vi "Autonomous Independent.vi"   [LabVIEW 2015]
doc: "This VI is called when autonomous begins, and will automatically be terminated when autonomous ends. You can carry out timed or sensor driven robot movement independently without needing to return to the caller."
uses:
  <vilib>/Rock Robotics/WPI/SafetyOutput/WPI_SafetyOutputConfigMenu.ctl
  <vilib>/Rock Robotics/Network Tables/NT Read String.vi
  <vilib>/Rock Robotics/WPI/Utilities/WPI_GetSetVariantRefNum.vi
  <vilib>/addons/control/pid/pid.llb/PID (DBL).vi
  <vilib>/Rock Robotics/WPI/Solenoid/Deprecated/WPI_SolenoidSetBool.vi
  Z navX/navX Library v2/navX Library v2.lvlib
  <vilib>/addons/control/pid/NI_PID_pid.lvlib
panel:
  # "Be sure to right-click and choose Data Operations>>Make Current Value default if you want to save the array values with the VI"
types:
  T1 = cluster{"proportional gain (Kc)":dbl, "integral time (Ti, min)":dbl, "derivative time (Td, min)":dbl}
  T2 = typedef "WPI_SafetyOutputConfigMenu.ctl" = enum16{"Enable", "Disable"}
  T3 = typedef "navX Library v2.lvlib/Z900_navX_DeviceTypeDef.ctl" = cluster{"Interface":cluster{"Protocol":T4, "Update Rate (4Hz-60Hz)":u8, "navX Open TypeDef":variant}, "Notify Packet":refnum<notifier>, "Loop VI Refnum":refnum<vi>, "Ready to Close Occurrence Refnum":refnum<k4>}
  T4 = typedef "navX Library v2.lvlib/Z900_navX_ProtocolTypeDef.ctl" = enum16{"SERIAL", "I2C", "SPI"}
  T5 = cluster{"LinearAcceleration X":dbl, "LinearAcceleration Y":dbl, "LinearAcceleration Z":dbl}
  T6 = cluster{"Velocity X":dbl, "Velocity Y":dbl, "Velocity Z":dbl, "Displacement X":dbl, "Displacement Y":dbl, "Displacement Z":dbl}
  T7 = typedef "WPI_RobotDriveDevRef.ctl" = cluster{"DevStatus":errorcluster, "Motors[]":T8[], "Square Inputs":bool, "Max Output":dbl}
  T8 = typedef "WPI_MotorControlDeviceRef.ctl" = cluster{"DeviceStatus":errorcluster, "Type":T9, "PWM":cluster{"PWM Channel":T10, "DeadBand":T11}, "CAN":cluster{"Device Number":u8, "Control Mode":T12, "Semaphore":T13, "Max Vout":dbl, "TalonSRX Control Mode":T14}, "Invert":bool}
  T9 = typedef "WPI_MotorControlType.ctl" = enum16{"PWM", "CAN", "CANTalonSRX"}
  T10 = typedef "FPGA_DIOPWMChannel.ctl" = enum8{"PWM 0", "PWM 1", "PWM 2", "PWM 3", "PWM 4", "PWM 5", "PWM 6", "PWM 7", "PWM 8", "PWM 9", "PWM MXP 0", "PWM MXP 1", "PWM MXP 2", "PWM MXP 3", "PWM MXP 4", "PWM MXP 5", "PWM MXP 6", "PWM MXP 7", "PWM MXP 8", "PWM MXP 9", "Invalid"}
  T11 = typedef "WPI_PWMDeadband.ctl" = cluster{"Name":string, "maxPositivePwm":i32, "minPositivePwm":i32, "centerPwm":i32, "maxNegativePwm":i32, "minNegativePwm":i32, "angularRange":u16}
  T12 = typedef "WPI_CANJaguar_ControlMode.ctl" = enum8{"Percent VBus", "Current", "Speed", "Position", "Voltage"}
  T13 = typedef "Semaphore RefNum" = refnum<k1>
  T14 = typedef "WPI_CANTalonSRX_APIControlMode.ctl" = enum8{"Percent VBus", "Speed", "Position", "Slave", "Unchanged / Invalid", "Voltage Compensation", "Current", "Motion Profile"}
  T15 = cluster{"Yaw":dbl, "Roll":dbl, "Pitch":dbl, "Heading":dbl, "Fused Heading":dbl}
  T16 = typedef "WPI_SolenoidDevRef.ctl" = cluster{"DevStatus":errorcluster, "Pneumatics Control Module":u8, "Forward Solenoid Channel":T17, "Reverse Solenoid Channel":T17}
  T17 = typedef "WPI_SolenoidChannel.ctl" = enum8{"Solenoid 0", "Solenoid 1", "Solenoid 2", "Solenoid 3", "Solenoid 4", "Solenoid 5", "Solenoid 6", "Solenoid 7", "Invalid"}
  T18 = typedef "WPI_CANTalonSRX_GlobalStatus.ctl" = cluster{"Applied Throttle":dbl, "Module Enabled":bool, "CAN Error":errorcluster, "Closed Loop Error":dbl, "Forward Limit Switch Closed":bool, "Reverse Limit Switch Closed":bool, "Sensor Position":dbl, "Sensor Velocity":dbl, "Current":dbl, "Sticky Fault - Over Temp":bool, "Sticky Fault - Under Voltage":bool, "Sticky Fault - Forward Limit":bool, "Sticky Fault - Reverse Limit":bool, "Sticky Fault - Forward Soft Limit":bool, "Sticky Fault - Reverse Soft Limit":bool, "Brake is Enabled":bool, "Encoder Position":dbl, "Encoder Velocity":dbl, "Encoder Index Count":dbl, "Encoder A Pin State":bool, "Encoder B Pin State":bool, "Encoder Index Pin State":bool, "Analog In":dbl, "Analog In Velocity":dbl, "Temperature (C)":dbl, "Battery Voltage":dbl, "Control 5 Is Supported":bool, "Current Profile Slot Select":dbl, "Pos Div 8":bool, "Vel Div 4":bool, "Pulse Width Position":i32, "Pulse Width Velocity":i32, "Pulse Width Rise To Rise (us)":i32, "Pulse Width Rise To Fall (us)":i32, "Mot Prof Active Is Under Run":bool, "Mot Prof Active Has Under Run":bool, "Mot Prof Active Is Last":bool, "Mot Prof Active Velocity Only":bool, "Mot Prof Active Is Valid":bool, "Mot Prof Buffer Is Full":bool, "Mot Prof Active Profile Slot Select":i32, "Mot Prof NextID":i32, "Mot Prof Count":i32, "Mot Prof Active Velocity":dbl, "Mot Prof Active Position":dbl, "Mot Prof Output Enable":i32}
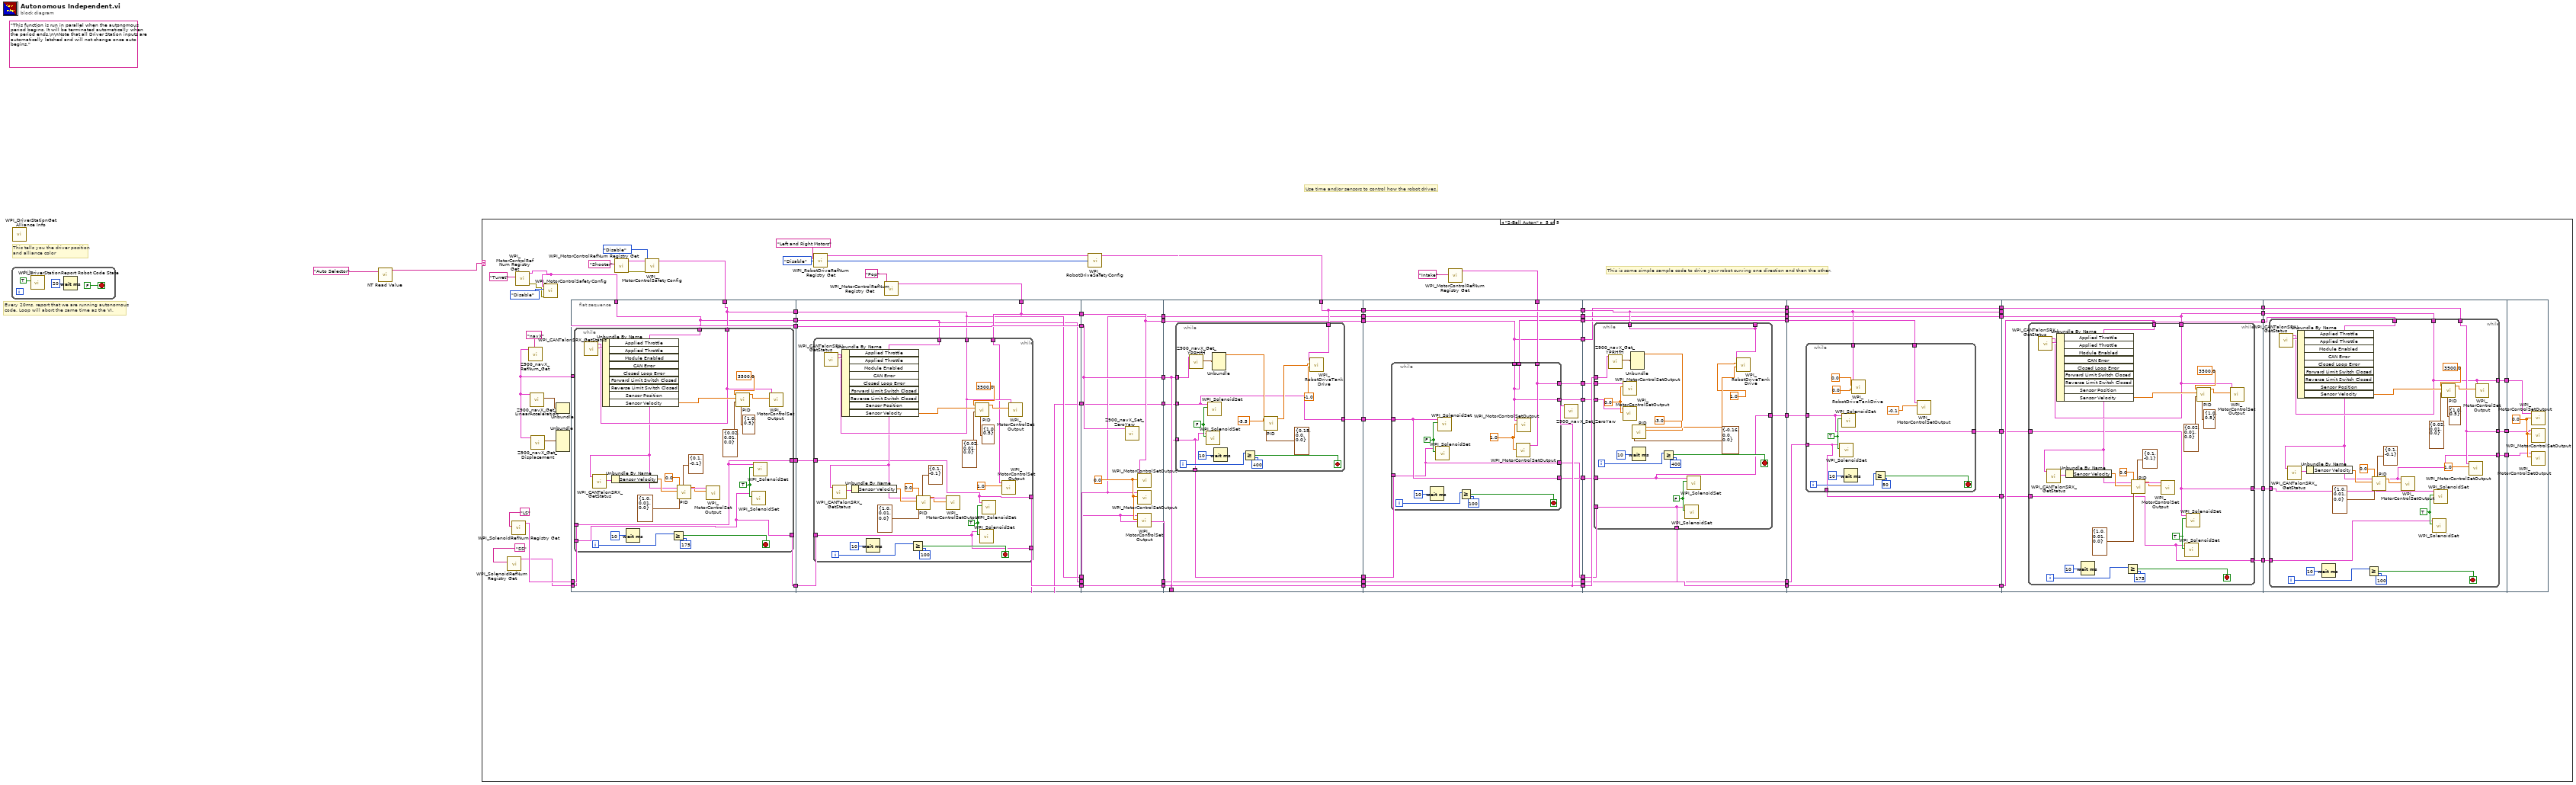
[diagram p0: block diagram]
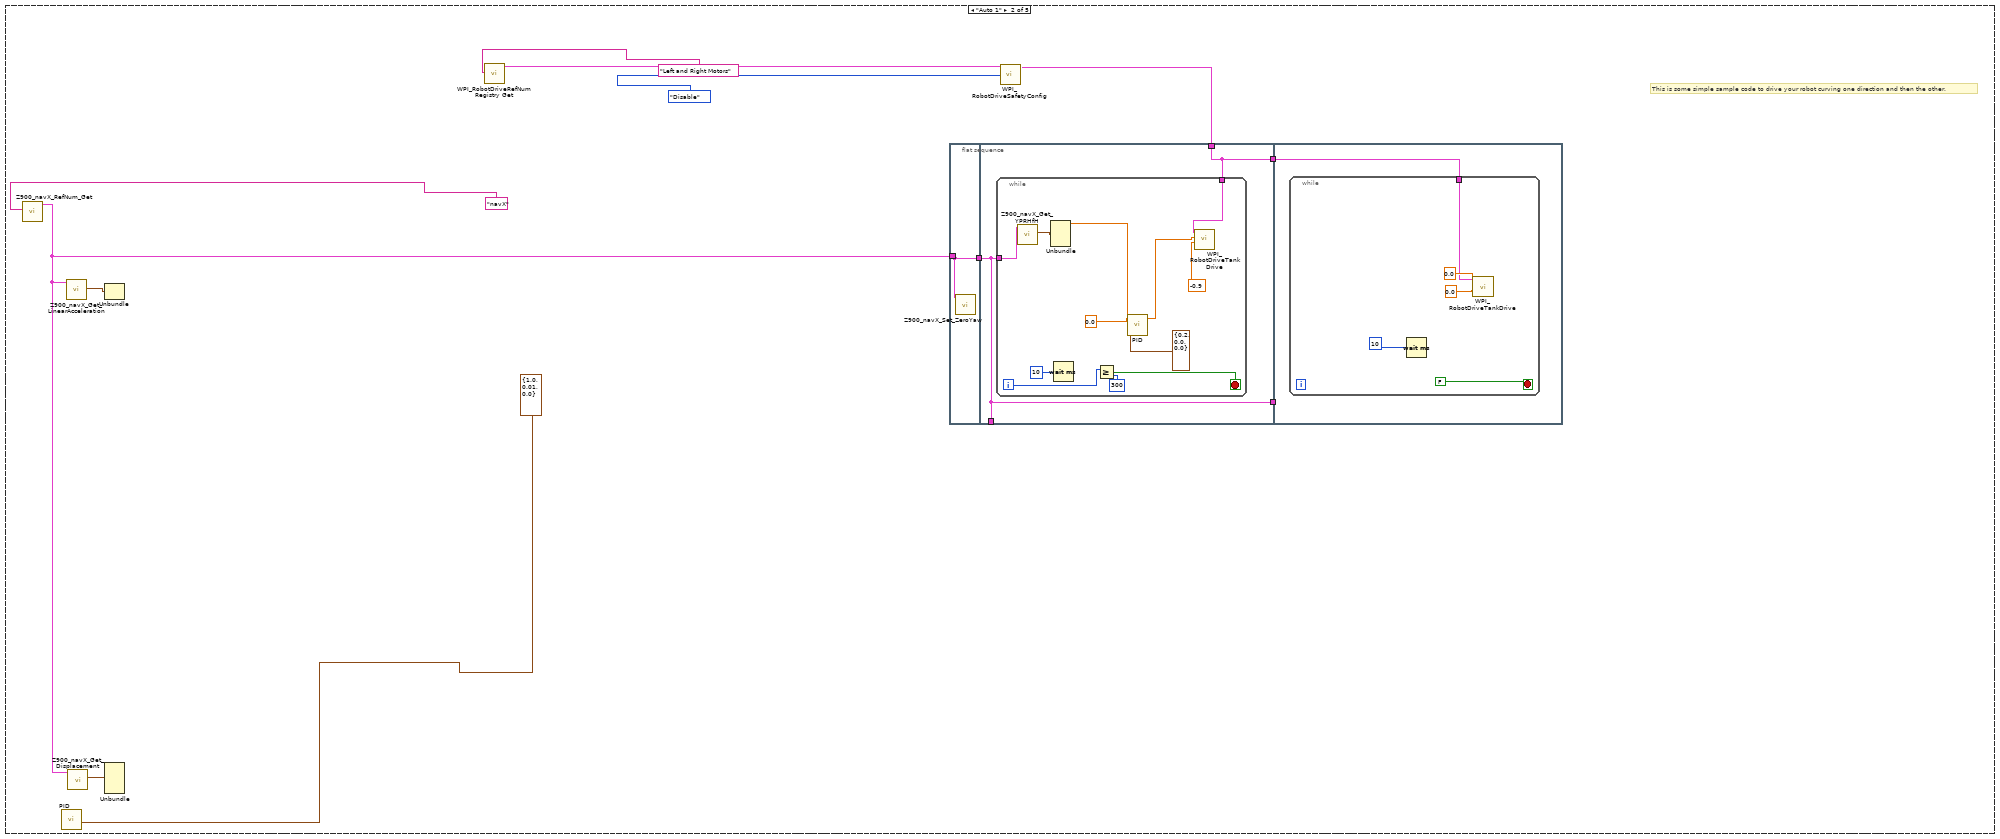
[diagram p3: hidden frame]
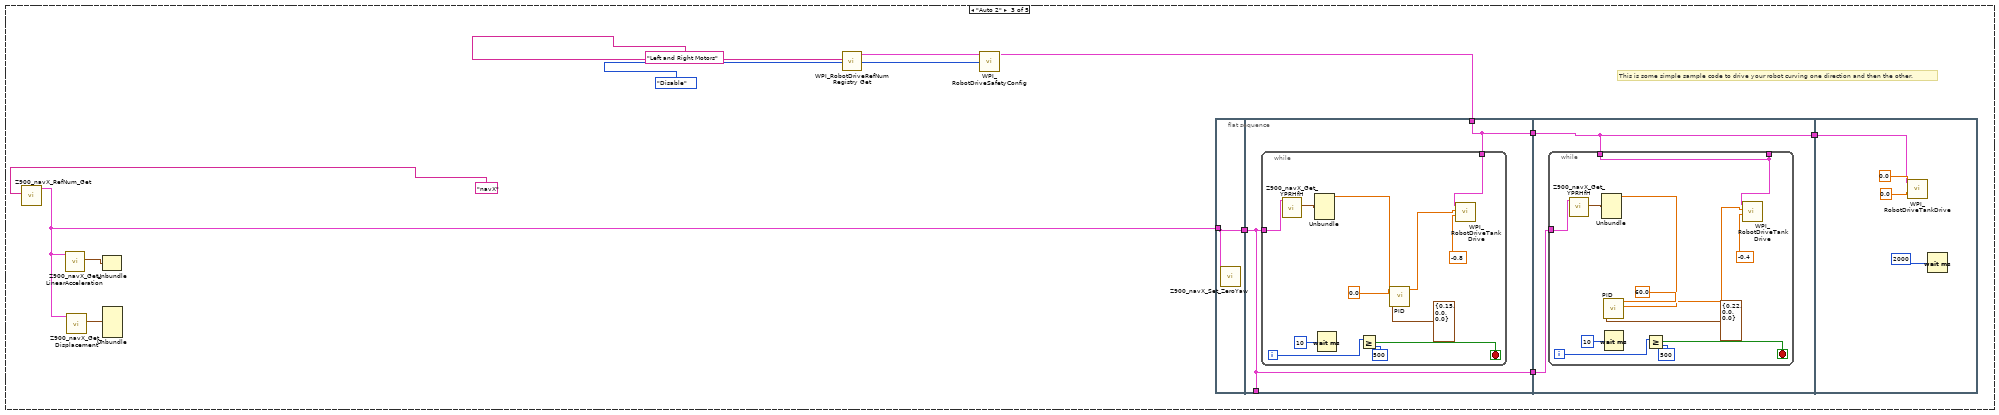
[diagram p4: hidden frame]
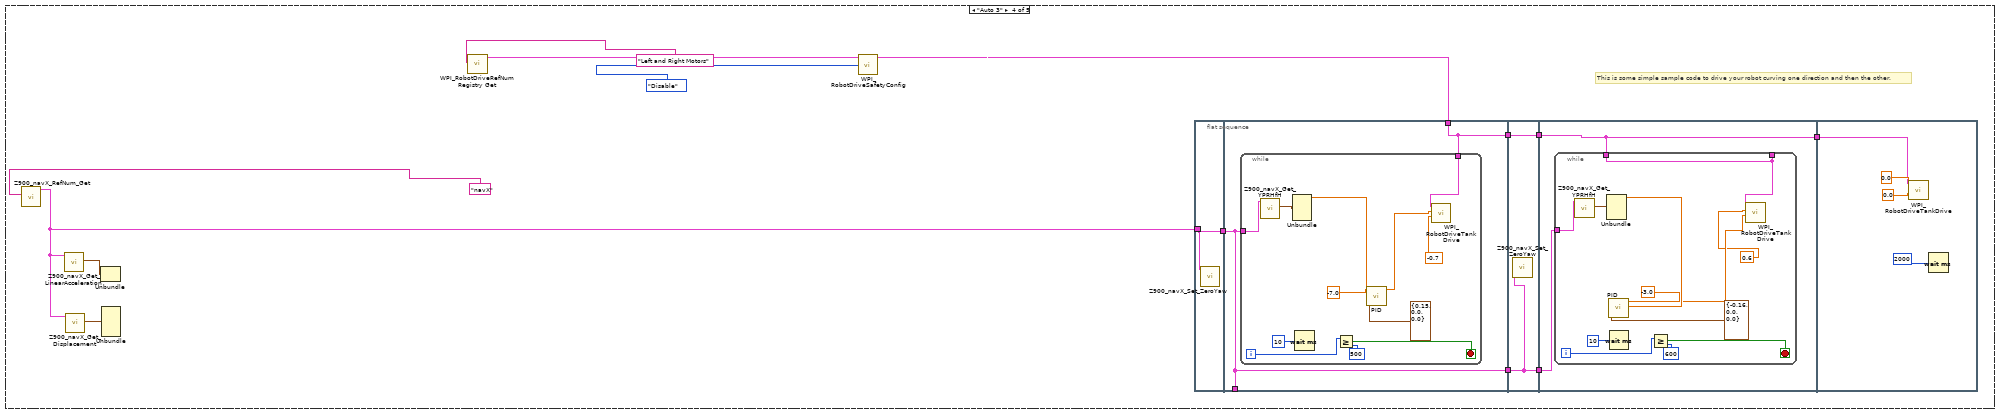
[diagram p5: hidden frame]
diagram:
  (unwired) "This function is run in parallel when the autonomous period begins. It will be terminated automatically when the period ends.\n\nNote that all Driver Station inputs are automatically latched and will not change once auto begins."
  # "Use time and/or sensors to control how the robot drives."
  # "Every 20ms, report that we are running autonomous\ncode. Loop will abort the same time as the VI."
  # "This tells you the driver position\nand alliance color"
  n1 = while {
    stop <- FALSE stop-if-true
    n2 = call <vilib>:"WPI_DriverStationReport Robot Code State.vi"("Autonomous"=TRUE) -> ()  [unwired: 10 in, 1 out]
    n3 = Wait (ms)(milliseconds to wait=u32 20) -> ()  [unwired: 1 out]
  }
  n4 = call <vilib>:"WPI_DriverStationGet Alliance Info.vi"() -> ()  [unwired: 12 out]
  n5 = call-poly <vilib>:"NT Read Value.vi"("Name"="Auto Selector") -> ("String"=w1:string)  [unwired: 9 in, 1 out]
  n6 = case shown="\"2-Ball Auton\"" w1 {
    frame Default {
      # "You can put your main auto here, or you can right-click on the case and make any\nother frame be the default case."
      # "This is the frame that will execute if no selection is made, or if it is not recognized"
    }
    frame "Auto 1" {
      # "This is some simple sample code to drive your robot curving one direction and then the other."
      n7 = call "Z900_navX_RefNum_Get.vi"("refnum name"="navX") -> ("navX Device"=w9:T3)  [unwired: 9 in, 1 out]
      n8 = call-poly <vilib>:"PID.vi"("PID gains"=T1 {"proportional gain (Kc)"=1.0, "integral time (Ti, min)"=0.01, "derivative time (Td, min)"=0.0}) -> ()  [unwired: 9 in, 2 out]
      n9 = call "Z900_navX_Get_LinearAcceleration.vi"("navX Device"=w9) -> ("Linear Acceleration"=w11:T5)  [unwired: 7 in, 3 out]
      n10 = call "Z900_navX_Get_Displacement.vi"("navX Device"=w9) -> ("Displacement"=w10:T6)  [unwired: 7 in, 3 out]
      n11 = Unbundle(w11) -> ()  [unwired: 3 out]
      n12 = Unbundle(w10) -> ()  [unwired: 6 out]
      n13 = call <vilib>:"WPI_RobotDriveRefNum Registry Get.vi"("refnum name"="Left and Right Motors") -> ("RobotDriveDevRef"=w14:T7)  [unwired: 9 in, 1 out]
      n14 = flat-sequence {
        tunnel: w9 -> [w18]
        tunnel: [w18] -> w7
        tunnel: w13 -> [w20]
        tunnel: [w20] -> w17
        tunnel: w7 -> [w19]
        tunnel: [w19] -> _
        tunnel: [w19] -> w6
        tunnel: w17 -> [w33]
        tunnel: w6 -> [_]
        frame #0 {
          n15 = call "Z900_navX_Set_ZeroYaw.vi"("navX Device"=w18) -> ()  [unwired: 9 in, 2 out]
        }
        frame #1 {
          n16 = while {
            tunnel: w20 -> [w29]
            tunnel: w19 -> [w24]
            i -> [w28]
            stop <- w26 stop-if-true
            n17 = call "Z900_navX_Get_YPRHfH.vi"("navX Device"=w24) -> ("YRPHfH"=w25:T15)  [unwired: 7 in, 3 out]
            n18 = Unbundle(w25) -> ("Yaw"=w21:dbl)  [unwired: 4 out]
            n19 = Wait (ms)(milliseconds to wait=10) -> ()  [unwired: 1 out]
            n20 = Greater Or Equal?(x=w28, y=300) -> (x >= y?=w26:bool)
            n21 = call-poly <vilib>:"PID.vi"("PID gains"=T1 {"proportional gain (Kc)"=0.2, "integral time (Ti, min)"=0.0, "derivative time (Td, min)"=0.0}, "process variable"=w21, "setpoint"=0.0) -> ("output"=w22:dbl)  [unwired: 7 in, 1 out]
            n22 = call <vilib>:"WPI_RobotDriveTankDrive.vi"("Right axis value"=-0.9, "Left axis value"=w22, "RobotDriveDevRef"=w29) -> ()  [unwired: 6 in, 3 out]
          }
        }
        frame #2 {
          n23 = while {
            tunnel: w33 -> [w35]
            stop <- FALSE stop-if-true
            n24 = Wait (ms)(milliseconds to wait=10) -> ()  [unwired: 1 out]
            n25 = call <vilib>:"WPI_RobotDriveTankDrive.vi"("Right axis value"=0.0, "Left axis value"=0.0, "RobotDriveDevRef"=w35) -> ()  [unwired: 6 in, 3 out]
          }
        }
      }
      n26 = call <vilib>:"WPI_RobotDriveSafetyConfig.vi"("mode"=WPI_SafetyOutputConfigMenu."Disable", "RobotDriveDevRef"=w14) -> ("RobotDriveDevRef"=w13:T7)  [unwired: 8 in, 1 out]
    }
    frame "Auto 2" {
      # "This is some simple sample code to drive your robot curving one direction and then the other."
      n27 = call "Z900_navX_RefNum_Get.vi"("refnum name"="navX") -> ("navX Device"=w39:T3)  [unwired: 9 in, 1 out]
      n28 = call "Z900_navX_Get_LinearAcceleration.vi"("navX Device"=w39) -> ("Linear Acceleration"=w41:T5)  [unwired: 7 in, 3 out]
      n29 = call "Z900_navX_Get_Displacement.vi"("navX Device"=w39) -> ("Displacement"=w40:T6)  [unwired: 7 in, 3 out]
      n30 = Unbundle(w41) -> ()  [unwired: 3 out]
      n31 = Unbundle(w40) -> ()  [unwired: 6 out]
      n32 = call <vilib>:"WPI_RobotDriveRefNum Registry Get.vi"("refnum name"="Left and Right Motors") -> ("RobotDriveDevRef"=w44:T7)  [unwired: 9 in, 1 out]
      n33 = call <vilib>:"WPI_RobotDriveSafetyConfig.vi"("mode"=WPI_SafetyOutputConfigMenu."Disable", "RobotDriveDevRef"=w44) -> ("RobotDriveDevRef"=w43:T7)  [unwired: 8 in, 1 out]
      n34 = flat-sequence {
        tunnel: w39 -> [w51]
        tunnel: [w51] -> w50
        tunnel: w43 -> [w53]
        tunnel: [w53] -> w49
        tunnel: w50 -> [w52]
        tunnel: [w52] -> _
        tunnel: [w52] -> w48
        tunnel: w49 -> [w67]
        tunnel: [w67] -> w47
        tunnel: w48 -> [w66]
        tunnel: w47 -> [w80]
        frame #0 {
          n35 = call "Z900_navX_Set_ZeroYaw.vi"("navX Device"=w51) -> ()  [unwired: 9 in, 2 out]
        }
        frame #1 {
          n36 = while {
            tunnel: w53 -> [w62]
            tunnel: w52 -> [w57]
            i -> [w61]
            stop <- w59 stop-if-true
            n37 = call "Z900_navX_Get_YPRHfH.vi"("navX Device"=w57) -> ("YRPHfH"=w58:T15)  [unwired: 7 in, 3 out]
            n38 = Unbundle(w58) -> ("Yaw"=w54:dbl)  [unwired: 4 out]
            n39 = Wait (ms)(milliseconds to wait=10) -> ()  [unwired: 1 out]
            n40 = Greater Or Equal?(x=w61, y=500) -> (x >= y?=w59:bool)
            n41 = call-poly <vilib>:"PID.vi"("PID gains"=T1 {"proportional gain (Kc)"=0.15, "integral time (Ti, min)"=0.0, "derivative time (Td, min)"=0.0}, "process variable"=w54, "setpoint"=0.0) -> ("output"=w55:dbl)  [unwired: 7 in, 1 out]
            n42 = call <vilib>:"WPI_RobotDriveTankDrive.vi"("Right axis value"=-0.8, "Left axis value"=w55, "RobotDriveDevRef"=w62) -> ()  [unwired: 6 in, 3 out]
          }
        }
        frame #2 {
          n43 = while {
            tunnel: [w68] -> _
            tunnel: w66 -> [w71]
            tunnel: w67 -> [w68]
            i -> [w76]
            stop <- w74 stop-if-true
            n44 = call "Z900_navX_Get_YPRHfH.vi"("navX Device"=w71) -> ("YRPHfH"=w73:T15)  [unwired: 7 in, 3 out]
            n45 = Unbundle(w73) -> ("Yaw"=w72:dbl)  [unwired: 4 out]
            n46 = call-poly <vilib>:"PID.vi"("PID gains"=T1 {"proportional gain (Kc)"=0.22, "integral time (Ti, min)"=0.0, "derivative time (Td, min)"=0.0}, "process variable"=w72, "setpoint"=60.0) -> ("output"=w69:dbl)  [unwired: 7 in, 1 out]
            n47 = Wait (ms)(milliseconds to wait=10) -> ()  [unwired: 1 out]
            n48 = Greater Or Equal?(x=w76, y=500) -> (x >= y?=w74:bool)
            n49 = call <vilib>:"WPI_RobotDriveTankDrive.vi"("Right axis value"=-0.4, "Left axis value"=w69, "RobotDriveDevRef"=w68) -> ()  [unwired: 6 in, 3 out]
          }
        }
        frame #3 {
          n50 = call <vilib>:"WPI_RobotDriveTankDrive.vi"("Right axis value"=0.0, "Left axis value"=0.0, "RobotDriveDevRef"=w80) -> ()  [unwired: 6 in, 3 out]
          n51 = Wait (ms)(milliseconds to wait=2000) -> ()  [unwired: 1 out]
        }
      }
    }
    frame "Auto 3" {
      # "This is some simple sample code to drive your robot curving one direction and then the other."
      n52 = call "Z900_navX_RefNum_Get.vi"("refnum name"="navX") -> ("navX Device"=w88:T3)  [unwired: 9 in, 1 out]
      n53 = call "Z900_navX_Get_LinearAcceleration.vi"("navX Device"=w88) -> ("Linear Acceleration"=w90:T5)  [unwired: 7 in, 3 out]
      n54 = call "Z900_navX_Get_Displacement.vi"("navX Device"=w88) -> ("Displacement"=w89:T6)  [unwired: 7 in, 3 out]
      n55 = Unbundle(w90) -> ()  [unwired: 3 out]
      n56 = Unbundle(w89) -> ()  [unwired: 6 out]
      n57 = call <vilib>:"WPI_RobotDriveRefNum Registry Get.vi"("refnum name"="Left and Right Motors") -> ("RobotDriveDevRef"=w93:T7)  [unwired: 9 in, 1 out]
      n58 = call <vilib>:"WPI_RobotDriveSafetyConfig.vi"("mode"=WPI_SafetyOutputConfigMenu."Disable", "RobotDriveDevRef"=w93) -> ("RobotDriveDevRef"=w92:T7)  [unwired: 8 in, 1 out]
      n59 = flat-sequence {
        tunnel: w88 -> [w98]
        tunnel: [w98] -> w97
        tunnel: w92 -> [w100]
        tunnel: [w100] -> w87
        tunnel: w97 -> [w99]
        tunnel: [w99] -> _
        tunnel: [w99] -> w85
        tunnel: w87 -> [w114]
        tunnel: [w114] -> w86
        tunnel: w85 -> [w113]
        tunnel: [w113] -> w84
        tunnel: w86 -> [w116]
        tunnel: [w116] -> w96
        tunnel: w84 -> [w115]
        tunnel: w96 -> [w129]
        frame #0 {
          n60 = call "Z900_navX_Set_ZeroYaw.vi"("navX Device"=w98) -> ()  [unwired: 9 in, 2 out]
        }
        frame #1 {
          n61 = while {
            tunnel: w100 -> [w109]
            tunnel: w99 -> [w104]
            i -> [w108]
            stop <- w106 stop-if-true
            n62 = call "Z900_navX_Get_YPRHfH.vi"("navX Device"=w104) -> ("YRPHfH"=w105:T15)  [unwired: 7 in, 3 out]
            n63 = Unbundle(w105) -> ("Yaw"=w101:dbl)  [unwired: 4 out]
            n64 = Wait (ms)(milliseconds to wait=10) -> ()  [unwired: 1 out]
            n65 = Greater Or Equal?(x=w108, y=500) -> (x >= y?=w106:bool)
            n66 = call-poly <vilib>:"PID.vi"("PID gains"=T1 {"proportional gain (Kc)"=0.15, "integral time (Ti, min)"=0.0, "derivative time (Td, min)"=0.0}, "process variable"=w101, "setpoint"=-7.0) -> ("output"=w102:dbl)  [unwired: 7 in, 1 out]
            n67 = call <vilib>:"WPI_RobotDriveTankDrive.vi"("Right axis value"=-0.7, "Left axis value"=w102, "RobotDriveDevRef"=w109) -> ()  [unwired: 6 in, 3 out]
          }
        }
        frame #2 {
          n68 = call "Z900_navX_Set_ZeroYaw.vi"("navX Device"=w113) -> ()  [unwired: 9 in, 2 out]
        }
        frame #3 {
          n69 = while {
            tunnel: [w119] -> _
            tunnel: w115 -> [w120]
            tunnel: w116 -> [w119]
            i -> [w125]
            stop <- w123 stop-if-true
            n70 = call "Z900_navX_Get_YPRHfH.vi"("navX Device"=w120) -> ("YRPHfH"=w122:T15)  [unwired: 7 in, 3 out]
            n71 = Unbundle(w122) -> ("Yaw"=w121:dbl)  [unwired: 4 out]
            n72 = call-poly <vilib>:"PID.vi"("PID gains"=T1 {"proportional gain (Kc)"=-0.16, "integral time (Ti, min)"=0.0, "derivative time (Td, min)"=0.0}, "process variable"=w121, "setpoint"=-3.0) -> ("output"=w118:dbl)  [unwired: 7 in, 1 out]
            n73 = Wait (ms)(milliseconds to wait=10) -> ()  [unwired: 1 out]
            n74 = Greater Or Equal?(x=w125, y=600) -> (x >= y?=w123:bool)
            n75 = call <vilib>:"WPI_RobotDriveTankDrive.vi"("Right axis value"=w118, "Left axis value"=0.6, "RobotDriveDevRef"=w119) -> ()  [unwired: 6 in, 3 out]
          }
        }
        frame #4 {
          n76 = call <vilib>:"WPI_RobotDriveTankDrive.vi"("Right axis value"=0.0, "Left axis value"=0.0, "RobotDriveDevRef"=w129) -> ()  [unwired: 6 in, 3 out]
          n77 = Wait (ms)(milliseconds to wait=2000) -> ()  [unwired: 1 out]
        }
      }
    }
    frame "2-Ball Auton" {
      # "This is some simple sample code to drive your robot curving one direction and then the other."
      n78 = call <vilib>:"WPI_SolenoidRefNum Registry Get.vi"("refnum name"="SS") -> ("SolenoidDevRef"=w149:T16)  [unwired: 9 in, 1 out]
      n79 = call <vilib>:"WPI_SolenoidRefNum Registry Get.vi"("refnum name"="LS") -> ("SolenoidDevRef"=w150:T16)  [unwired: 9 in, 1 out]
      n80 = call <vilib>:"WPI_MotorControlRefNum Registry Get.vi"("refnum name"="Turret") -> ("error out"=w187:errorcluster, "MotorControlDevRef"=w189:T8)  [unwired: 9 in]
      n81 = call "Z900_navX_RefNum_Get.vi"("refnum name"="navX") -> ("navX Device"=w204:T3)  [unwired: 9 in, 1 out]
      n82 = call "Z900_navX_Get_LinearAcceleration.vi"("navX Device"=w204) -> ("Linear Acceleration"=w206:T5)  [unwired: 7 in, 3 out]
      n83 = call "Z900_navX_Get_Displacement.vi"("navX Device"=w204) -> ("Displacement"=w205:T6)  [unwired: 7 in, 3 out]
      n84 = call <vilib>:"WPI_MotorControlSafetyConfig.vi"("error in (no error)"=w187, "mode"=WPI_SafetyOutputConfigMenu."Disable", "MotorControlDevRef"=w189) -> ()  [unwired: 7 in, 2 out]
      n85 = Unbundle(w206) -> ()  [unwired: 3 out]
      n86 = Unbundle(w205) -> ()  [unwired: 6 out]
      n87 = flat-sequence {
        tunnel: w204 -> [w219]
        tunnel: [w219] -> w198
        tunnel: w193 -> [w218]
        tunnel: w189 -> [w217]
        tunnel: [w218] -> w191
        tunnel: [w217] -> w190
        tunnel: w150 -> [w216]
        tunnel: w149 -> [w215]
        tunnel: [w214] -> w148
        tunnel: [w213] -> w147
        tunnel: [w248] -> w199
        tunnel: w198 -> [w248]
        tunnel: w191 -> [w246]
        tunnel: w190 -> [w245]
        tunnel: w185 -> [w247]
        tunnel: [w247] -> w184
        tunnel: [w246] -> w183
        tunnel: [w245] -> w182
        tunnel: w148 -> [w244]
        tunnel: w147 -> [w243]
        tunnel: [w242] -> w145
        tunnel: [w241] -> w143
        tunnel: [w278] -> w212
        tunnel: w199 -> [w278]
        tunnel: w184 -> [w276]
        tunnel: w183 -> [w275]
        tunnel: w182 -> [w274]
        tunnel: [w276] -> w179
        tunnel: [w275] -> w167
        tunnel: [w274] -> w162
        tunnel: [w273] -> w146
        tunnel: w145 -> [w273]
        tunnel: [w272] -> w144
        tunnel: w143 -> [w272]
        tunnel: w208 -> [w287]
        tunnel: [w287] -> w203
        tunnel: w212 -> [w286]
        tunnel: [w286] -> _
        tunnel: [w286] -> w201
        tunnel: [w285] -> w180
        tunnel: w179 -> [w285]
        tunnel: [w284] -> w168
        tunnel: w167 -> [w284]
        tunnel: [w283] -> w163
        tunnel: w162 -> [w283]
        tunnel: w146 -> [w282]
        tunnel: w144 -> [w281]
        tunnel: [w280] -> w142
        tunnel: [w279] -> w141
        tunnel: w203 -> [w315]
        tunnel: [w315] -> w202
        tunnel: w201 -> [w314]
        tunnel: [w314] -> w200
        tunnel: w180 -> [w307]
        tunnel: w178 -> [w313]
        tunnel: [w312] -> w174
        tunnel: [w311] -> w173
        tunnel: [w310] -> w172
        tunnel: [w309] -> w169
        tunnel: w168 -> [w309]
        tunnel: [w308] -> w164
        tunnel: w163 -> [w308]
        tunnel: [w307] -> w156
        tunnel: w142 -> [w306]
        tunnel: w141 -> [w305]
        tunnel: [w304] -> w140
        tunnel: [w303] -> w139
        tunnel: w202 -> [w337]
        tunnel: [w337] -> w177
        tunnel: w200 -> [w336]
        tunnel: [w335] -> w175
        tunnel: w174 -> [w335]
        tunnel: w173 -> [w334]
        tunnel: w172 -> [w333]
        tunnel: [w332] -> w170
        tunnel: w169 -> [w332]
        tunnel: [w331] -> w165
        tunnel: w164 -> [w331]
        tunnel: [w330] -> w157
        tunnel: w156 -> [w330]
        tunnel: w140 -> [w329]
        tunnel: w139 -> [w328]
        tunnel: [w327] -> w138
        tunnel: [w326] -> w137
        tunnel: w177 -> [w363]
        tunnel: [w363] -> w176
        tunnel: w175 -> [w364]
        tunnel: [w362] -> w171
        tunnel: w170 -> [w362]
        tunnel: [w361] -> w166
        tunnel: w165 -> [w361]
        tunnel: [w360] -> w158
        tunnel: w157 -> [w360]
        tunnel: w138 -> [w359]
        tunnel: w137 -> [w358]
        tunnel: [w357] -> w136
        tunnel: [w356] -> w135
        tunnel: w176 -> [_]
        tunnel: w171 -> [w382]
        tunnel: w166 -> [w383]
        tunnel: [w383] -> w161
        tunnel: [w382] -> w160
        tunnel: [w381] -> w159
        tunnel: w158 -> [w381]
        tunnel: w136 -> [w380]
        tunnel: w135 -> [w379]
        tunnel: [w378] -> w134
        tunnel: [w377] -> w133
        tunnel: w161 -> [w412]
        tunnel: w160 -> [w411]
        tunnel: w159 -> [w410]
        tunnel: [w409] -> w155
        tunnel: [w408] -> w154
        tunnel: [w407] -> w153
        tunnel: w134 -> [w406]
        tunnel: w133 -> [w405]
        tunnel: w155 -> [w438]
        tunnel: w154 -> [w437]
        tunnel: w153 -> [w436]
        frame #0 {
          n88 = while {
            tunnel: w218 -> [w231]
            tunnel: w217 -> [w224]
            tunnel: w216 -> [w220]
            tunnel: w215 -> [w221]
            tunnel: [w221] -> w214
            tunnel: [w220] -> w213
            i -> [w239]
            stop <- w237 stop-if-true
            w222 = TRUE
            n89 = call <vilib>:"WPI_CANTalonSRX_GetStatus.vi"("CAN Talon SRX Ref"=w231) -> ("Talon SRX Status"=w233:T18)  [unwired: 8 in, 2 out]
            n90 = call <vilib>:"WPI_CANTalonSRX_GetStatus.vi"("CAN Talon SRX Ref"=w224) -> ("Talon SRX Status"=w229:T18)  [unwired: 8 in, 2 out]
            n91 = Unbundle By Name(w233) -> ("Sensor Velocity"=w235:dbl)  [unwired: 8 out]
            n92 = Unbundle By Name(w229) -> ("Sensor Velocity"=w228:dbl)
            n93 = Wait (ms)(milliseconds to wait=10) -> ()  [unwired: 1 out]
            n94 = Greater Or Equal?(x=w239, y=175) -> (x >= y?=w237:bool)
            n95 = call-poly <vilib>:"PID.vi"("output range"=cluster{"output high":dbl, "output low":dbl} {"output high"=0.1, "output low"=-0.1}, "PID gains"=T1 {"proportional gain (Kc)"=1.0, "integral time (Ti, min)"=0.01, "derivative time (Td, min)"=0.0}, "process variable"=w228, "setpoint"=0.0) -> ("output"=w223:dbl)  [unwired: 6 in, 1 out]
            n96 = call <vilib>:"WPI_MotorControlSetOutput.vi"("Output"=w223, "MotorControlDevRef"=w224) -> ()  [unwired: 7 in, 3 out]
            n97 = call-poly <vilib>:"PID.vi"("output range"=cluster{"output high":dbl, "output low":dbl} {"output high"=1.0, "output low"=0.5}, "PID gains"=T1 {"proportional gain (Kc)"=0.02, "integral time (Ti, min)"=0.01, "derivative time (Td, min)"=0.0}, "process variable"=w235, "setpoint"=3500.0) -> ("output"=w234:dbl)  [unwired: 6 in, 1 out]
            n98 = call-poly <vilib>:"WPI_SolenoidSet.vi"("Value"=w222, "SolenoidDevRef"=w221) -> ()  [unwired: 1 in, 9 out]
            n99 = call-poly <vilib>:"WPI_SolenoidSet.vi"("Value"=w222, "SolenoidDevRef"=w220) -> ()  [unwired: 1 in, 9 out]
            n100 = call <vilib>:"WPI_MotorControlSetOutput.vi"("Output"=w234, "MotorControlDevRef"=w231) -> ()  [unwired: 7 in, 3 out]
          }
        }
        frame #1 {
          n101 = while {
            tunnel: w246 -> [w262]
            tunnel: w245 -> [w255]
            tunnel: w247 -> [w253]
            tunnel: w244 -> [w250]
            tunnel: w243 -> [w249]
            tunnel: [w250] -> w242
            tunnel: [w249] -> w241
            i -> [w270]
            stop <- w268 stop-if-true
            w251 = TRUE
            n102 = call <vilib>:"WPI_CANTalonSRX_GetStatus.vi"("CAN Talon SRX Ref"=w262) -> ("Talon SRX Status"=w264:T18)  [unwired: 8 in, 2 out]
            n103 = call <vilib>:"WPI_CANTalonSRX_GetStatus.vi"("CAN Talon SRX Ref"=w255) -> ("Talon SRX Status"=w260:T18)  [unwired: 8 in, 2 out]
            n104 = Unbundle By Name(w264) -> ("Sensor Velocity"=w266:dbl)  [unwired: 8 out]
            n105 = Unbundle By Name(w260) -> ("Sensor Velocity"=w259:dbl)
            n106 = Wait (ms)(milliseconds to wait=10) -> ()  [unwired: 1 out]
            n107 = Greater Or Equal?(x=w270, y=100) -> (x >= y?=w268:bool)
            n108 = call-poly <vilib>:"PID.vi"("output range"=cluster{"output high":dbl, "output low":dbl} {"output high"=0.1, "output low"=-0.1}, "PID gains"=T1 {"proportional gain (Kc)"=1.0, "integral time (Ti, min)"=0.01, "derivative time (Td, min)"=0.0}, "process variable"=w259, "setpoint"=0.0) -> ("output"=w254:dbl)  [unwired: 6 in, 1 out]
            n109 = call <vilib>:"WPI_MotorControlSetOutput.vi"("Output"=w254, "MotorControlDevRef"=w255) -> ()  [unwired: 7 in, 3 out]
            n110 = call-poly <vilib>:"PID.vi"("output range"=cluster{"output high":dbl, "output low":dbl} {"output high"=1.0, "output low"=0.5}, "PID gains"=T1 {"proportional gain (Kc)"=0.02, "integral time (Ti, min)"=0.01, "derivative time (Td, min)"=0.0}, "process variable"=w266, "setpoint"=3500.0) -> ("output"=w265:dbl)  [unwired: 6 in, 1 out]
            n111 = call-poly <vilib>:"WPI_SolenoidSet.vi"("Value"=w251, "SolenoidDevRef"=w250) -> ()  [unwired: 1 in, 9 out]
            n112 = call-poly <vilib>:"WPI_SolenoidSet.vi"("Value"=w251, "SolenoidDevRef"=w249) -> ()  [unwired: 1 in, 9 out]
            n113 = call <vilib>:"WPI_MotorControlSetOutput.vi"("Output"=1.0, "MotorControlDevRef"=w253) -> ()  [unwired: 7 in, 3 out]
            n114 = call <vilib>:"WPI_MotorControlSetOutput.vi"("Output"=w265, "MotorControlDevRef"=w262) -> ()  [unwired: 7 in, 3 out]
          }
        }
        frame #2 {
          w277 = 0.0
          n115 = call "Z900_navX_Set_ZeroYaw.vi"("navX Device"=w278) -> ()  [unwired: 9 in, 2 out]
          n116 = call <vilib>:"WPI_MotorControlSetOutput.vi"("Output"=w277, "MotorControlDevRef"=w274) -> ()  [unwired: 7 in, 3 out]
          n117 = call <vilib>:"WPI_MotorControlSetOutput.vi"("Output"=w277, "MotorControlDevRef"=w276) -> ()  [unwired: 7 in, 3 out]
          n118 = call <vilib>:"WPI_MotorControlSetOutput.vi"("Output"=w277, "MotorControlDevRef"=w275) -> ()  [unwired: 7 in, 3 out]
        }
        frame #3 {
          n119 = while {
            tunnel: w287 -> [w299]
            tunnel: w286 -> [w294]
            tunnel: w282 -> [w288]
            tunnel: w281 -> [w289]
            tunnel: [w289] -> w280
            tunnel: [w288] -> w279
            i -> [w298]
            stop <- w296 stop-if-true
            w290 = FALSE
            n120 = call "Z900_navX_Get_YPRHfH.vi"("navX Device"=w294) -> ("YRPHfH"=w295:T15)  [unwired: 7 in, 3 out]
            n121 = call-poly <vilib>:"WPI_SolenoidSet.vi"("Value"=w290, "SolenoidDevRef"=w288) -> ()  [unwired: 1 in, 9 out]
            n122 = call-poly <vilib>:"WPI_SolenoidSet.vi"("Value"=w290, "SolenoidDevRef"=w289) -> ()  [unwired: 1 in, 9 out]
            n123 = Unbundle(w295) -> ("Yaw"=w291:dbl)  [unwired: 4 out]
            n124 = Wait (ms)(milliseconds to wait=10) -> ()  [unwired: 1 out]
            n125 = Greater Or Equal?(x=w298, y=400) -> (x >= y?=w296:bool)
            n126 = call-poly <vilib>:"PID.vi"("PID gains"=T1 {"proportional gain (Kc)"=0.15, "integral time (Ti, min)"=0.0, "derivative time (Td, min)"=0.0}, "process variable"=w291, "setpoint"=-5.5) -> ("output"=w292:dbl)  [unwired: 7 in, 1 out]
            n127 = call <vilib>:"WPI_RobotDriveTankDrive.vi"("Right axis value"=-1.0, "Left axis value"=w292, "RobotDriveDevRef"=w299) -> ()  [unwired: 6 in, 3 out]
          }
        }
        frame #4 {
          n128 = while {
            tunnel: w307 -> [w319]
            tunnel: w313 -> [w320]
            tunnel: [w319] -> w312
            tunnel: [w320] -> w311
            tunnel: [w319] -> w310
            tunnel: w306 -> [w317]
            tunnel: w305 -> [w316]
            tunnel: [w317] -> w304
            tunnel: [w316] -> w303
            i -> [w324]
            stop <- w322 stop-if-true
            w318 = FALSE
            w321 = 1.0
            n129 = Wait (ms)(milliseconds to wait=10) -> ()  [unwired: 1 out]
            n130 = call-poly <vilib>:"WPI_SolenoidSet.vi"("Value"=w318, "SolenoidDevRef"=w316) -> ()  [unwired: 1 in, 9 out]
            n131 = call-poly <vilib>:"WPI_SolenoidSet.vi"("Value"=w318, "SolenoidDevRef"=w317) -> ()  [unwired: 1 in, 9 out]
            n132 = Greater Or Equal?(x=w324, y=100) -> (x >= y?=w322:bool)
            n133 = call <vilib>:"WPI_MotorControlSetOutput.vi"("Output"=w321, "MotorControlDevRef"=w320) -> ()  [unwired: 7 in, 3 out]
            n134 = call <vilib>:"WPI_MotorControlSetOutput.vi"("Output"=w321, "MotorControlDevRef"=w319) -> ()  [unwired: 7 in, 3 out]
          }
          n135 = call "Z900_navX_Set_ZeroYaw.vi"("navX Device"=w314) -> ()  [unwired: 9 in, 2 out]
        }
        frame #5 {
          n136 = while {
            tunnel: [w346] -> _
            tunnel: w336 -> [w347]
            tunnel: w337 -> [w346]
            tunnel: w334 -> [w342]
            tunnel: w333 -> [w341]
            tunnel: w329 -> [w339]
            tunnel: w328 -> [w338]
            tunnel: [w339] -> w327
            tunnel: [w338] -> w326
            i -> [w352]
            stop <- w350 stop-if-true
            w340 = FALSE
            w343 = 0.0
            n137 = call "Z900_navX_Get_YPRHfH.vi"("navX Device"=w347) -> ("YRPHfH"=w349:T15)  [unwired: 7 in, 3 out]
            n138 = call <vilib>:"WPI_MotorControlSetOutput.vi"("Output"=w343, "MotorControlDevRef"=w341) -> ()  [unwired: 7 in, 3 out]
            n139 = call <vilib>:"WPI_MotorControlSetOutput.vi"("Output"=w343, "MotorControlDevRef"=w342) -> ()  [unwired: 7 in, 3 out]
            n140 = Unbundle(w349) -> ("Yaw"=w348:dbl)  [unwired: 4 out]
            n141 = call-poly <vilib>:"PID.vi"("PID gains"=T1 {"proportional gain (Kc)"=-0.16, "integral time (Ti, min)"=0.0, "derivative time (Td, min)"=0.0}, "process variable"=w348, "setpoint"=-3.0) -> ("output"=w345:dbl)  [unwired: 7 in, 1 out]
            n142 = Wait (ms)(milliseconds to wait=10) -> ()  [unwired: 1 out]
            n143 = Greater Or Equal?(x=w352, y=400) -> (x >= y?=w350:bool)
            n144 = call-poly <vilib>:"WPI_SolenoidSet.vi"("Value"=w340, "SolenoidDevRef"=w338) -> ()  [unwired: 1 in, 9 out]
            n145 = call-poly <vilib>:"WPI_SolenoidSet.vi"("Value"=w340, "SolenoidDevRef"=w339) -> ()  [unwired: 1 in, 9 out]
            n146 = call <vilib>:"WPI_RobotDriveTankDrive.vi"("Right axis value"=w345, "Left axis value"=1.0, "RobotDriveDevRef"=w346) -> ()  [unwired: 6 in, 3 out]
          }
        }
        frame #6 {
          n147 = while {
            tunnel: w364 -> [w372]
            tunnel: w363 -> [w368]
            tunnel: w359 -> [w366]
            tunnel: w358 -> [w365]
            tunnel: [w366] -> w357
            tunnel: [w365] -> w356
            i -> [w375]
            stop <- w373 stop-if-true
            w367 = TRUE
            n148 = call-poly <vilib>:"WPI_SolenoidSet.vi"("Value"=w367, "SolenoidDevRef"=w365) -> ()  [unwired: 1 in, 9 out]
            n149 = call-poly <vilib>:"WPI_SolenoidSet.vi"("Value"=w367, "SolenoidDevRef"=w366) -> ()  [unwired: 1 in, 9 out]
            n150 = Wait (ms)(milliseconds to wait=10) -> ()  [unwired: 1 out]
            n151 = call <vilib>:"WPI_RobotDriveTankDrive.vi"("Right axis value"=0.0, "Left axis value"=0.0, "RobotDriveDevRef"=w368) -> ()  [unwired: 6 in, 3 out]
            n152 = Greater Or Equal?(x=w375, y=50) -> (x >= y?=w373:bool)
            n153 = call <vilib>:"WPI_MotorControlSetOutput.vi"("Output"=-0.1, "MotorControlDevRef"=w372) -> ()  [unwired: 7 in, 3 out]
          }
        }
        frame #7 {
          n154 = while {
            tunnel: w382 -> [w395]
            tunnel: w383 -> [w388]
            tunnel: w380 -> [w385]
            tunnel: w379 -> [w384]
            tunnel: [w385] -> w378
            tunnel: [w384] -> w377
            i -> [w403]
            stop <- w401 stop-if-true
            w386 = TRUE
            n155 = call <vilib>:"WPI_CANTalonSRX_GetStatus.vi"("CAN Talon SRX Ref"=w395) -> ("Talon SRX Status"=w397:T18)  [unwired: 8 in, 2 out]
            n156 = call <vilib>:"WPI_CANTalonSRX_GetStatus.vi"("CAN Talon SRX Ref"=w388) -> ("Talon SRX Status"=w393:T18)  [unwired: 8 in, 2 out]
            n157 = Unbundle By Name(w397) -> ("Sensor Velocity"=w399:dbl)  [unwired: 8 out]
            n158 = Unbundle By Name(w393) -> ("Sensor Velocity"=w392:dbl)
            n159 = Wait (ms)(milliseconds to wait=10) -> ()  [unwired: 1 out]
            n160 = Greater Or Equal?(x=w403, y=175) -> (x >= y?=w401:bool)
            n161 = call-poly <vilib>:"PID.vi"("output range"=cluster{"output high":dbl, "output low":dbl} {"output high"=0.1, "output low"=-0.1}, "PID gains"=T1 {"proportional gain (Kc)"=1.0, "integral time (Ti, min)"=0.01, "derivative time (Td, min)"=0.0}, "process variable"=w392, "setpoint"=0.0) -> ("output"=w387:dbl)  [unwired: 6 in, 1 out]
            n162 = call <vilib>:"WPI_MotorControlSetOutput.vi"("Output"=w387, "MotorControlDevRef"=w388) -> ()  [unwired: 7 in, 3 out]
            n163 = call-poly <vilib>:"WPI_SolenoidSet.vi"("Value"=w386, "SolenoidDevRef"=w384) -> ()  [unwired: 1 in, 9 out]
            n164 = call-poly <vilib>:"WPI_SolenoidSet.vi"("Value"=w386, "SolenoidDevRef"=w385) -> ()  [unwired: 1 in, 9 out]
            n165 = call-poly <vilib>:"PID.vi"("output range"=cluster{"output high":dbl, "output low":dbl} {"output high"=1.0, "output low"=0.5}, "PID gains"=T1 {"proportional gain (Kc)"=0.02, "integral time (Ti, min)"=0.01, "derivative time (Td, min)"=0.0}, "process variable"=w399, "setpoint"=3500.0) -> ("output"=w398:dbl)  [unwired: 6 in, 1 out]
            n166 = call <vilib>:"WPI_MotorControlSetOutput.vi"("Output"=w398, "MotorControlDevRef"=w395) -> ()  [unwired: 7 in, 3 out]
          }
        }
        frame #8 {
          n167 = while {
            tunnel: w411 -> [w417]
            tunnel: w412 -> [w416]
            tunnel: w410 -> [w418]
            tunnel: [w418] -> w409
            tunnel: [w417] -> w408
            tunnel: [w416] -> w407
            tunnel: w406 -> [w414]
            tunnel: w405 -> [w413]
            i -> [w434]
            stop <- w432 stop-if-true
            w415 = TRUE
            n168 = call <vilib>:"WPI_CANTalonSRX_GetStatus.vi"("CAN Talon SRX Ref"=w417) -> ("Talon SRX Status"=w428:T18)  [unwired: 8 in, 2 out]
            n169 = call <vilib>:"WPI_CANTalonSRX_GetStatus.vi"("CAN Talon SRX Ref"=w416) -> ("Talon SRX Status"=w425:T18)  [unwired: 8 in, 2 out]
            n170 = Unbundle By Name(w428) -> ("Sensor Velocity"=w430:dbl)  [unwired: 8 out]
            n171 = Unbundle By Name(w425) -> ("Sensor Velocity"=w424:dbl)
            n172 = Wait (ms)(milliseconds to wait=10) -> ()  [unwired: 1 out]
            n173 = Greater Or Equal?(x=w434, y=100) -> (x >= y?=w432:bool)
            n174 = call-poly <vilib>:"PID.vi"("output range"=cluster{"output high":dbl, "output low":dbl} {"output high"=0.1, "output low"=-0.1}, "PID gains"=T1 {"proportional gain (Kc)"=1.0, "integral time (Ti, min)"=0.01, "derivative time (Td, min)"=0.0}, "process variable"=w424, "setpoint"=0.0) -> ("output"=w420:dbl)  [unwired: 6 in, 1 out]
            n175 = call <vilib>:"WPI_MotorControlSetOutput.vi"("Output"=w420, "MotorControlDevRef"=w416) -> ()  [unwired: 7 in, 3 out]
            n176 = call-poly <vilib>:"WPI_SolenoidSet.vi"("Value"=w415, "SolenoidDevRef"=w413) -> ()  [unwired: 1 in, 9 out]
            n177 = call-poly <vilib>:"WPI_SolenoidSet.vi"("Value"=w415, "SolenoidDevRef"=w414) -> ()  [unwired: 1 in, 9 out]
            n178 = call-poly <vilib>:"PID.vi"("output range"=cluster{"output high":dbl, "output low":dbl} {"output high"=1.0, "output low"=0.5}, "PID gains"=T1 {"proportional gain (Kc)"=0.02, "integral time (Ti, min)"=0.01, "derivative time (Td, min)"=0.0}, "process variable"=w430, "setpoint"=3500.0) -> ("output"=w429:dbl)  [unwired: 6 in, 1 out]
            n179 = call <vilib>:"WPI_MotorControlSetOutput.vi"("Output"=1.0, "MotorControlDevRef"=w418) -> ()  [unwired: 7 in, 3 out]
            n180 = call <vilib>:"WPI_MotorControlSetOutput.vi"("Output"=w429, "MotorControlDevRef"=w417) -> ()  [unwired: 7 in, 3 out]
          }
        }
        frame #9 {
          w439 = 0.0
          n181 = call <vilib>:"WPI_MotorControlSetOutput.vi"("Output"=w439, "MotorControlDevRef"=w436) -> ()  [unwired: 7 in, 3 out]
          n182 = call <vilib>:"WPI_MotorControlSetOutput.vi"("Output"=w439, "MotorControlDevRef"=w437) -> ()  [unwired: 7 in, 3 out]
          n183 = call <vilib>:"WPI_MotorControlSetOutput.vi"("Output"=w439, "MotorControlDevRef"=w438) -> ()  [unwired: 7 in, 3 out]
        }
      }
      n184 = call <vilib>:"WPI_MotorControlRefNum Registry Get.vi"("refnum name"="Shooter") -> ("error out"=w196:errorcluster, "MotorControlDevRef"=w195:T8)  [unwired: 9 in]
      n185 = call <vilib>:"WPI_MotorControlSafetyConfig.vi"("error in (no error)"=w196, "mode"=WPI_SafetyOutputConfigMenu."Disable", "MotorControlDevRef"=w195) -> ("MotorControlDevRef"=w193:T8)  [unwired: 7 in, 1 out]
      n186 = call <vilib>:"WPI_RobotDriveRefNum Registry Get.vi"("refnum name"="Left and Right Motors") -> ("RobotDriveDevRef"=w209:T7)  [unwired: 9 in, 1 out]
      n187 = call <vilib>:"WPI_MotorControlRefNum Registry Get.vi"("refnum name"="Pop") -> ("MotorControlDevRef"=w185:T8)  [unwired: 9 in, 1 out]
      n188 = call <vilib>:"WPI_RobotDriveSafetyConfig.vi"("mode"=WPI_SafetyOutputConfigMenu."Disable", "RobotDriveDevRef"=w209) -> ("RobotDriveDevRef"=w208:T7)  [unwired: 8 in, 1 out]
      n189 = call <vilib>:"WPI_MotorControlRefNum Registry Get.vi"("refnum name"="Intake") -> ("MotorControlDevRef"=w178:T8)  [unwired: 9 in, 1 out]
    }
  }
